vi "Get_FPGASimIO_Channel Data_5734.vi"(7 "Channel Name":string="Channel0", 8 "Error In":errorcluster) -> (0 "Error Out":errorcluster, 2 "Data":i16)   [LabVIEW 2012]
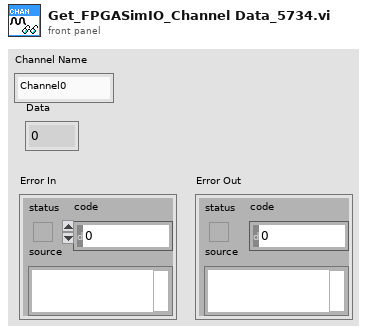
[diagram p1: front panel]
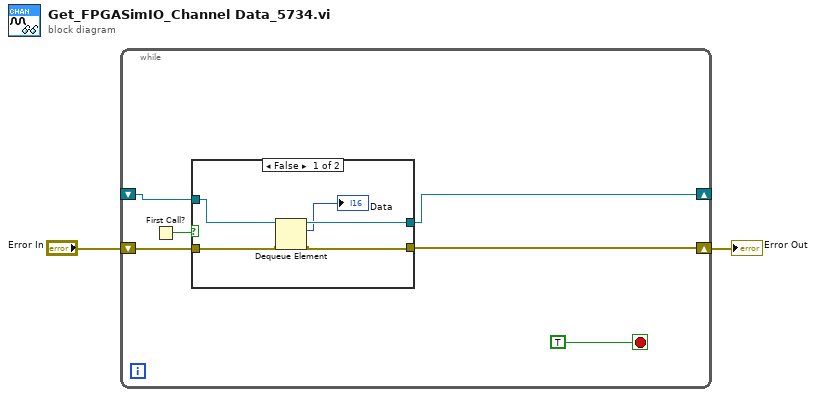
[diagram p0: block diagram]
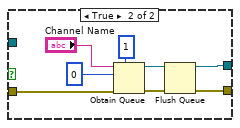
[diagram p2: hidden frame]
diagram:
  n1 = while {
    shift-right: [w7] -> w1
    shift-left: "Error In" -> [w5]
    shift-right: [w8] -> _
    shift-left: _ -> [w3]
    stop <- TRUE ("stop") stop-if-true
    n2 = First Call?() -> (First Call?: T/F=w6:bool)
    n3 = case shown="False" w6 {
      tunnel: [w12 w15] -> w8
      tunnel: [w10 w14] -> w7
      tunnel: w3 -> [w13 _]
      tunnel: w5 -> [w11 w20]
      frame False {
        n4 = Dequeue Element(queue=w13, error in (no error)=w11) -> (queue out=w12:refnum<queue>, element=→"Data":i16, error out=w10:errorcluster)  [unwired: 1 in, 1 out]
      }
      frame True {
        n5 = Obtain Queue(max queue size (-1, unlimited)=1, name (unnamed)="Channel Name", element data type=i16 0, error in (no error)=w20) -> (queue out=w16:refnum<queue>, error out=w17:errorcluster)  [unwired: 1 in, 1 out]
        n6 = Flush Queue(queue=w16, error in (no error)=w17) -> (queue out=w15:refnum<queue>, error out=w14:errorcluster)  [unwired: 1 out]
      }
    }
  }
  "Error Out" <- w1
